vi "General_Get Parent.vi"(8 "Error In (no Error)":errorcluster, 9 "Generations Back (1:parent)":i32=1, 11 "Get Ref? (t)":bool=TRUE) -> (0 "Error Out":errorcluster, 1 "Parent Vi Name Out":string, 3 "VI Refnum Out":refnum<vi>)   [LabVIEW 2009]
doc: "Get a reference to the current VI's Parrent"
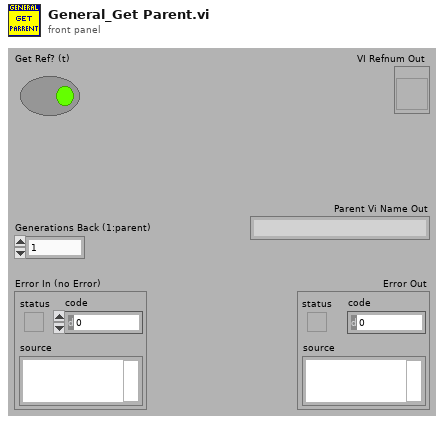
[diagram p1: front panel]
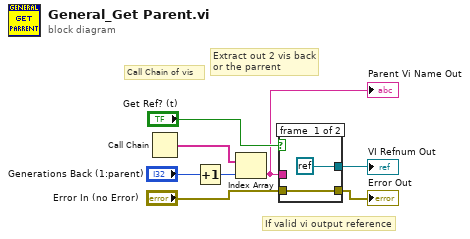
[diagram p0: block diagram]
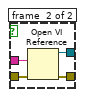
[diagram p2: hidden frame]
diagram:
  # "If valid vi output reference"
  # "Extract out 2 vis back\nor the parrent"
  # "Call Chain of vis"
  n1 = Call Chain() -> (call chain=w4:string[])
  n2 = Increment(x="Generations Back (1:parent)") -> (x+1=w1:i32)
  n3 = Index Array(array=w4, index=w1) -> (element=w6:string)
  "Parent Vi Name Out" <- w6
  n4 = case shown="True" "Get Ref? (t)" {
    tunnel: [refnum<k0> refnum w14] -> w2
    tunnel: [w9 w13] -> w3
    tunnel: w6 -> [_ w12]
    tunnel: "Error In (no Error)" -> [w9 w11]
    frame #0 {
    }
    frame #1 {
      n5 = Open VI Reference(vi path=w12, error in (no error)=w11) -> (vi reference=w14:refnum<vi>, error out=w13:errorcluster)  [unwired: 4 in]
    }
  }
  "Error Out" <- w3
  "VI Refnum Out" <- w2
